vi "Plotter_Competition_Main.vi"() -> ()   [LabVIEW 2014]
doc: "Buggy_Competition Main.vi\nv4.0\nCode fior Jan 2012\n\nModified by D.Readman 1/12/2011 to 5/1/2012 \n- Replaced shift registers with FGV's.\n- Latched Switch function added.\n- Digital filtering on encoder inputs added."
uses:
  Controls/Plotter States.ctl
  <vilib>/Platform/TimedLoop/XDataNode/timing_clust.ctl
  <vilib>/Platform/TimedLoop/XDataNode/nitl_modes.ctl
  <vilib>/Platform/TimedLoop/XDataNode/wakeup.ctl
  <vilib>/FPGAPlugInAG/myRIO-1900/niLvFpga_Open_myRIO-1900.vi
  <vilib>/rvi/interface/nirviOpenFPGA/nirviOpenFPGA.xnode
  FPGA Bitfiles/Buggycompetition_FPGATarget2_AeroBuggyFPGA_9DbUQD1BP7s.lvbitx
  FPGA/FPGA.vi
  <vilib>/Platform/TimedLoop/XDataNode/XDataNode.xnode
  <vilib>/Platform/TimedLoop/XDataNode/XDNodeRunTimeDep.lvlib
panel:
  out "Array 2":i32[][](array[numeric])
  out "M2 desired":i32
  out "M1 desired":i32
  out "m2 current":i16
  out "M1 current":i16
  out "Array":dbl[][](array[numeric])
  out "Finished Late? [i-1]":bool
  in  "Sample interval":u32=100000
  in  "MWidth":i64=4
  out "Current State":T1
  out "Switch B":bool
  out "Switch A":bool
  in  "Enc. Filter":i16=2 min=0 step=1
  out "Switches Latched":cluster{"Switch A GN":bool, "Switch B BL":bool}
  in  "Terminate":bool
  out "Error Display":errorcluster
  in  "Reset Button":bool
  # "Impeccable Plotter Controller"
  # "Switches"
  # "Admin controls - Do not alter"
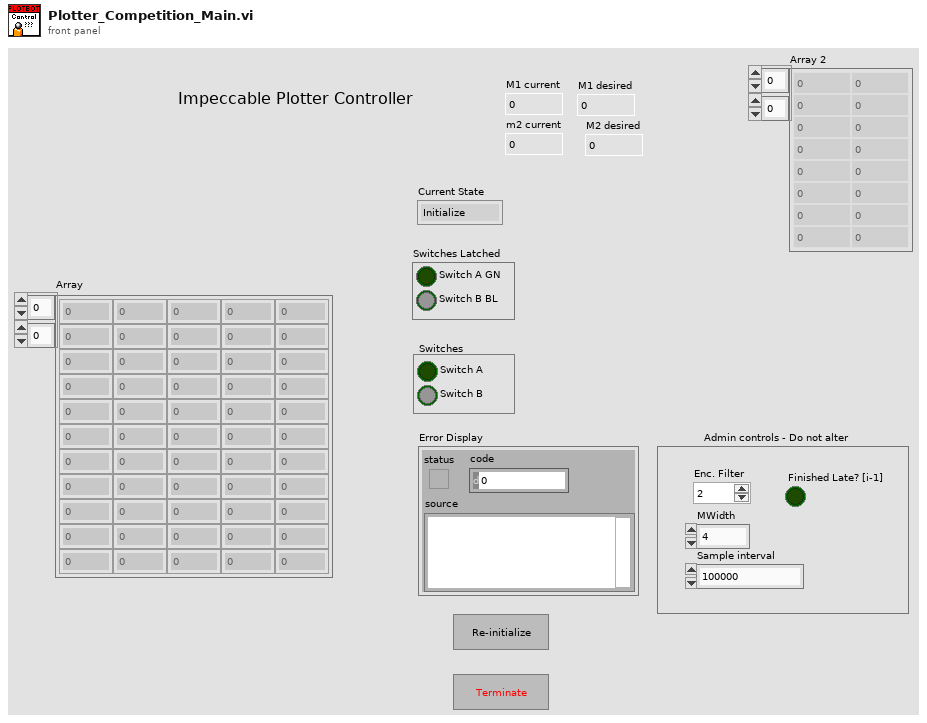
[diagram p1: front panel]
types:
  T1 = typedef "Plotter States.ctl" = enum16{"Initialize", "Run", "Stop"}
  T2 = cluster{"Data":dbl[], "Operation":enum16{"New folder/file", "Create file", "Record", "Close"}, "File name":string}
  T3 = typedef "XDNodeRunTimeDep.lvlib/timing_clust.ctl" = cluster{"Expected End [f-1]":u64, "Actual End [f-1]":u64, "Finished Late? [f-1]":bool, "Expected End [i-1]":u64, "Actual End [i-1]":u64, "Finished Late? [i-1]":bool, "Expected Start [i]":u64, "Actual Start [i]":u64, "Expected Start [f]":u64, "Actual Start [f]":u64, "Source Name":string, "Structure Name":string, "Period":i64, "Deadline":i64, "Offset":i64, "Start":i64, "Priority":i32, "Timeout":i32, "Mode":T4, "Wakeup Reason":T5, "Error":errorcluster, "Source Type":string, "Secondary Source Type":string, "Global End Time":u64, "Global Start Time":u64, "Frame Duration":u64, "Iteration Duration":u64, "Assigned CPU":i32, "I/O Scan Engine Mode":u32}
  T4 = typedef "XDNodeRunTimeDep.lvlib/nitl_modes.ctl" = enum32{"No Change", "Process missed periods, maintain original phase", "Discard missed periods, maintain original phase", "Process missed periods, ignore original phase", "Discard missed periods, ignore original phase"}
  T5 = typedef "XDNodeRunTimeDep.lvlib/wakeup.ctl" = enum32{"Normal", "Aborted", "Asynchronous wakeup", "Timing source error", "Timed loop error", "Timeout"}
  T6 = enum16{"New folder/file", "Create file", "Record", "Close"}
  T7 = cluster{"appended array":dbl[], "Operation":enum16{"New folder/file", "Create file", "Record", "Close"}, string}
  T8 = cluster{dbl[], "Operation":enum16{"New folder/file", "Create file", "Record", "Close"}, string}
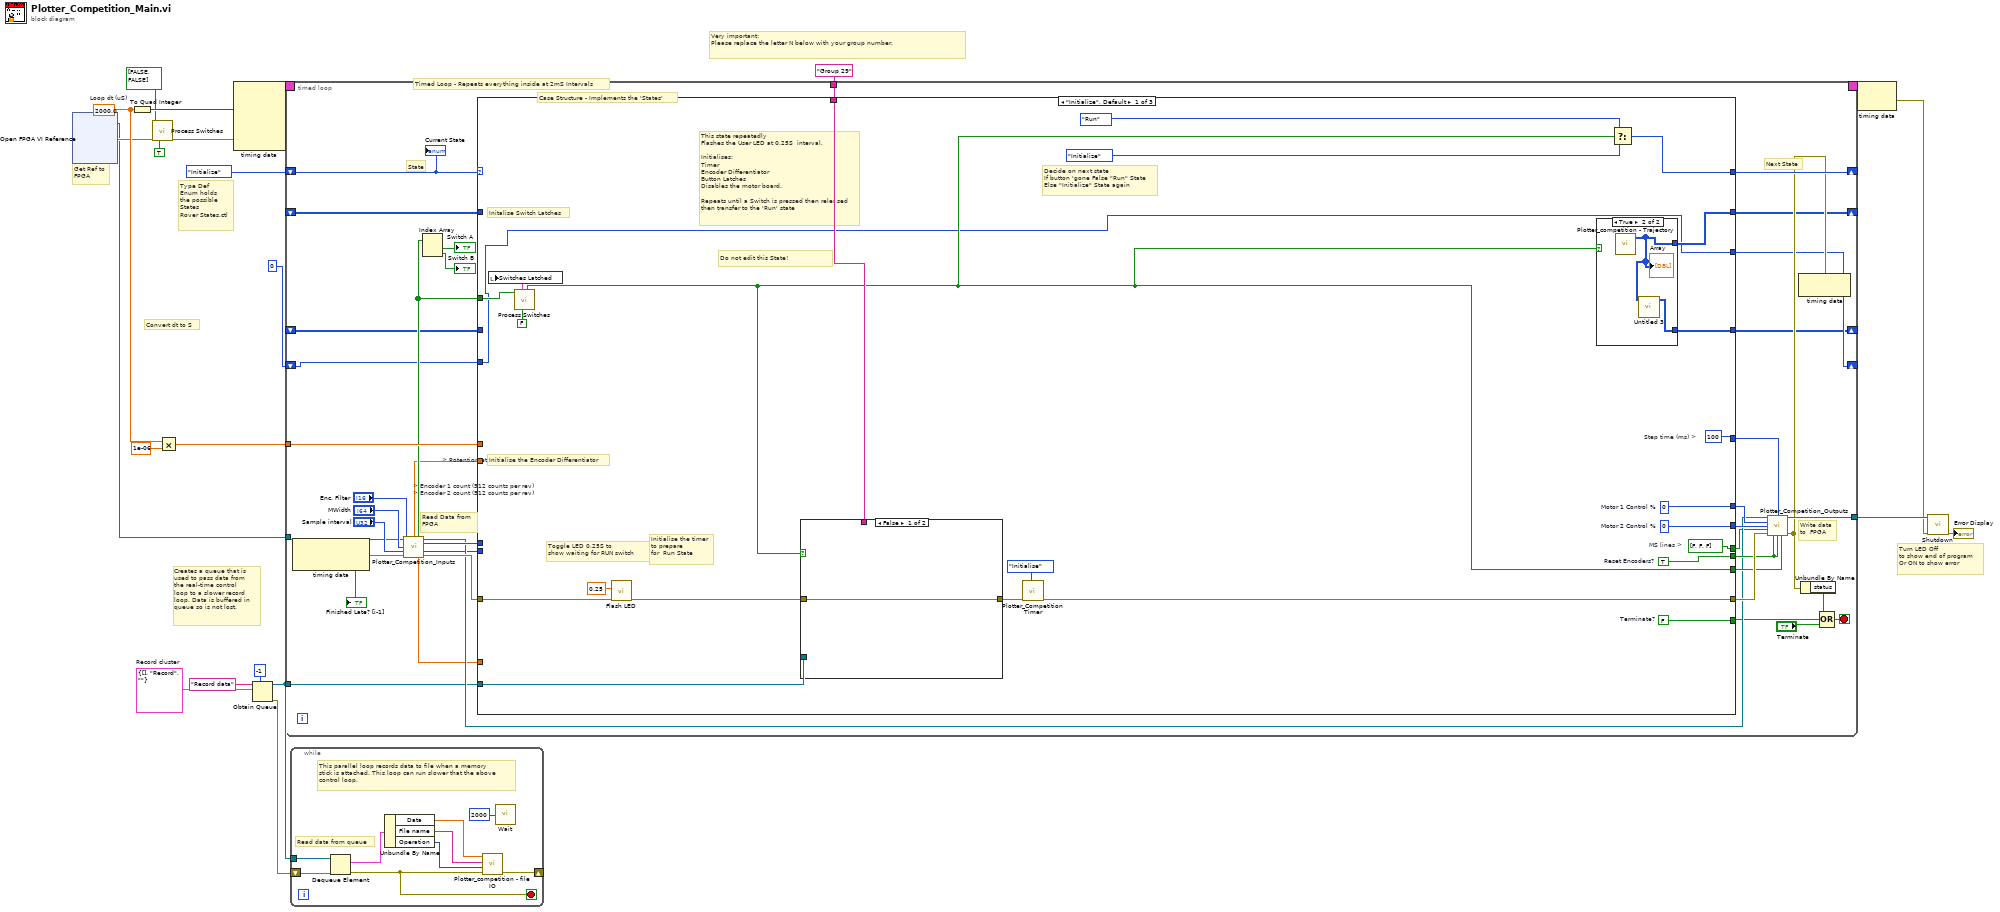
[diagram p0: block diagram]
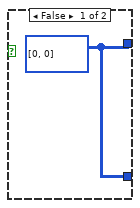
[diagram p2: hidden frame]
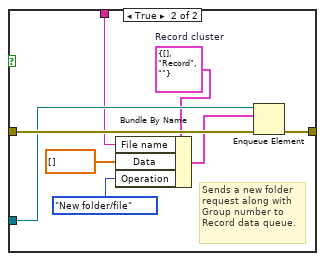
[diagram p3: hidden frame]
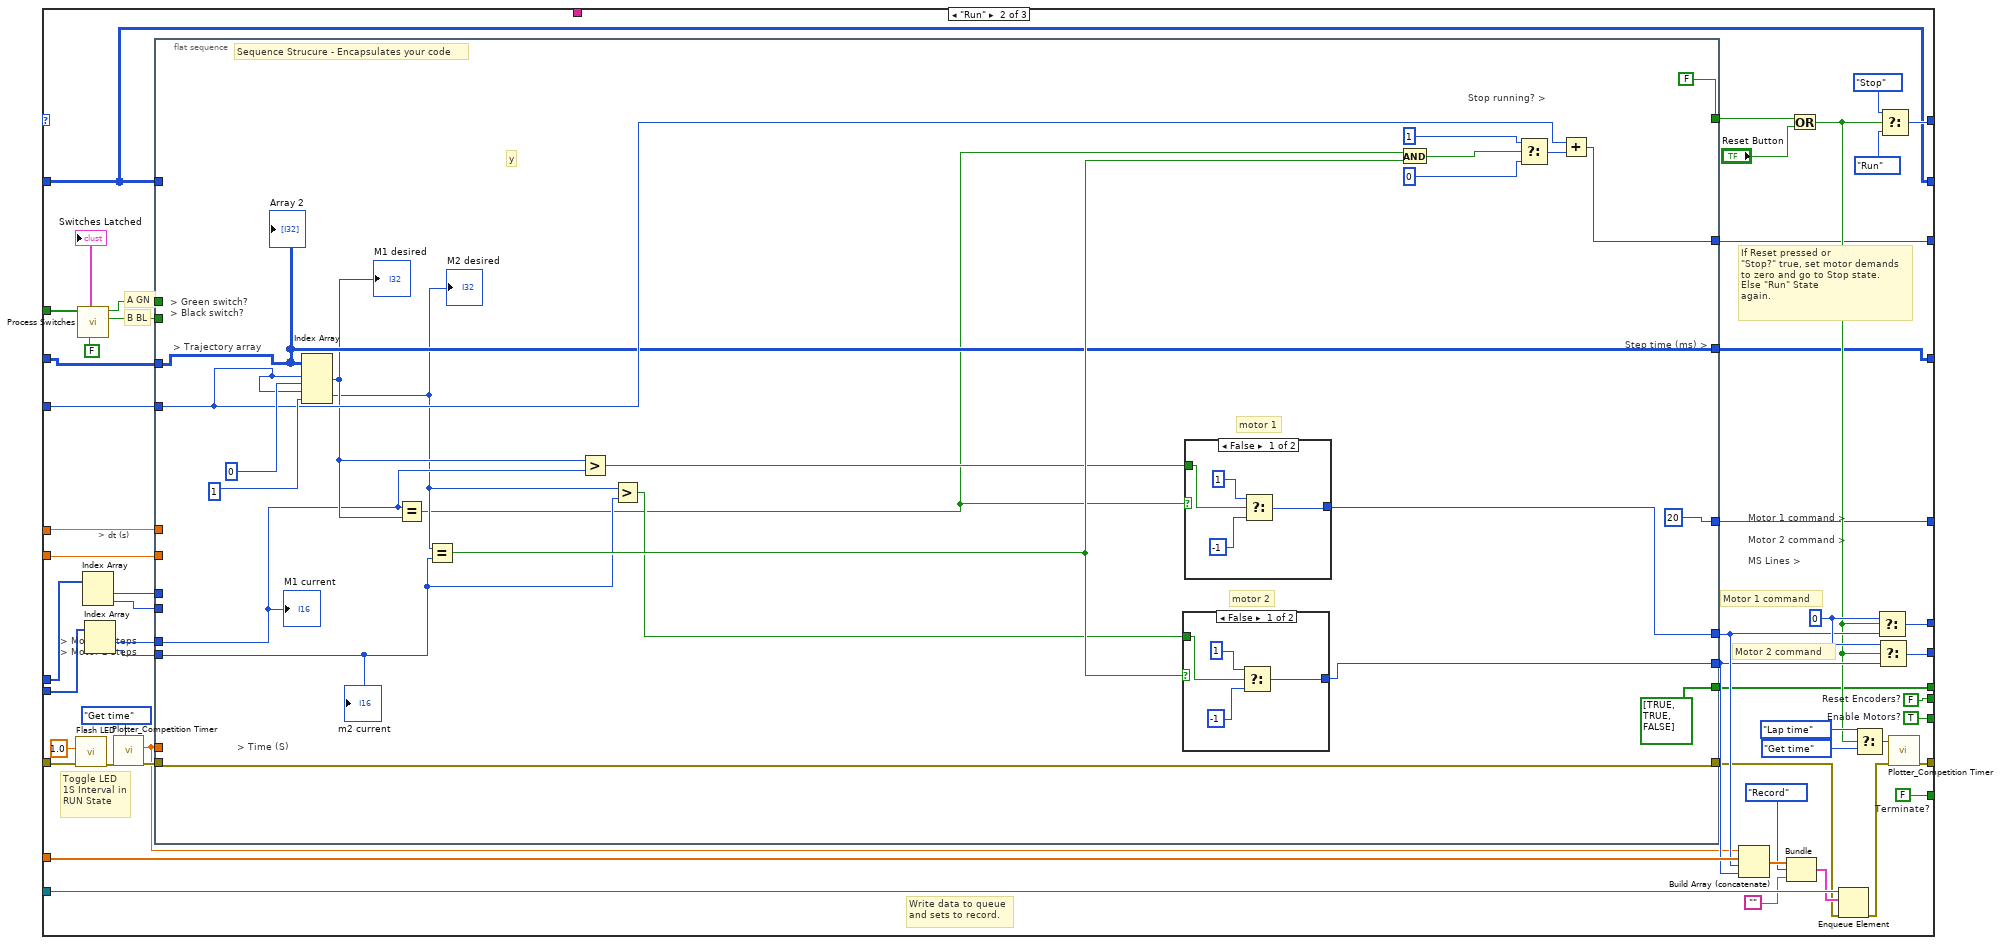
[diagram p4: hidden frame]
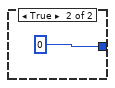
[diagram p5: hidden frame]
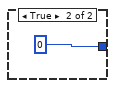
[diagram p6: hidden frame]
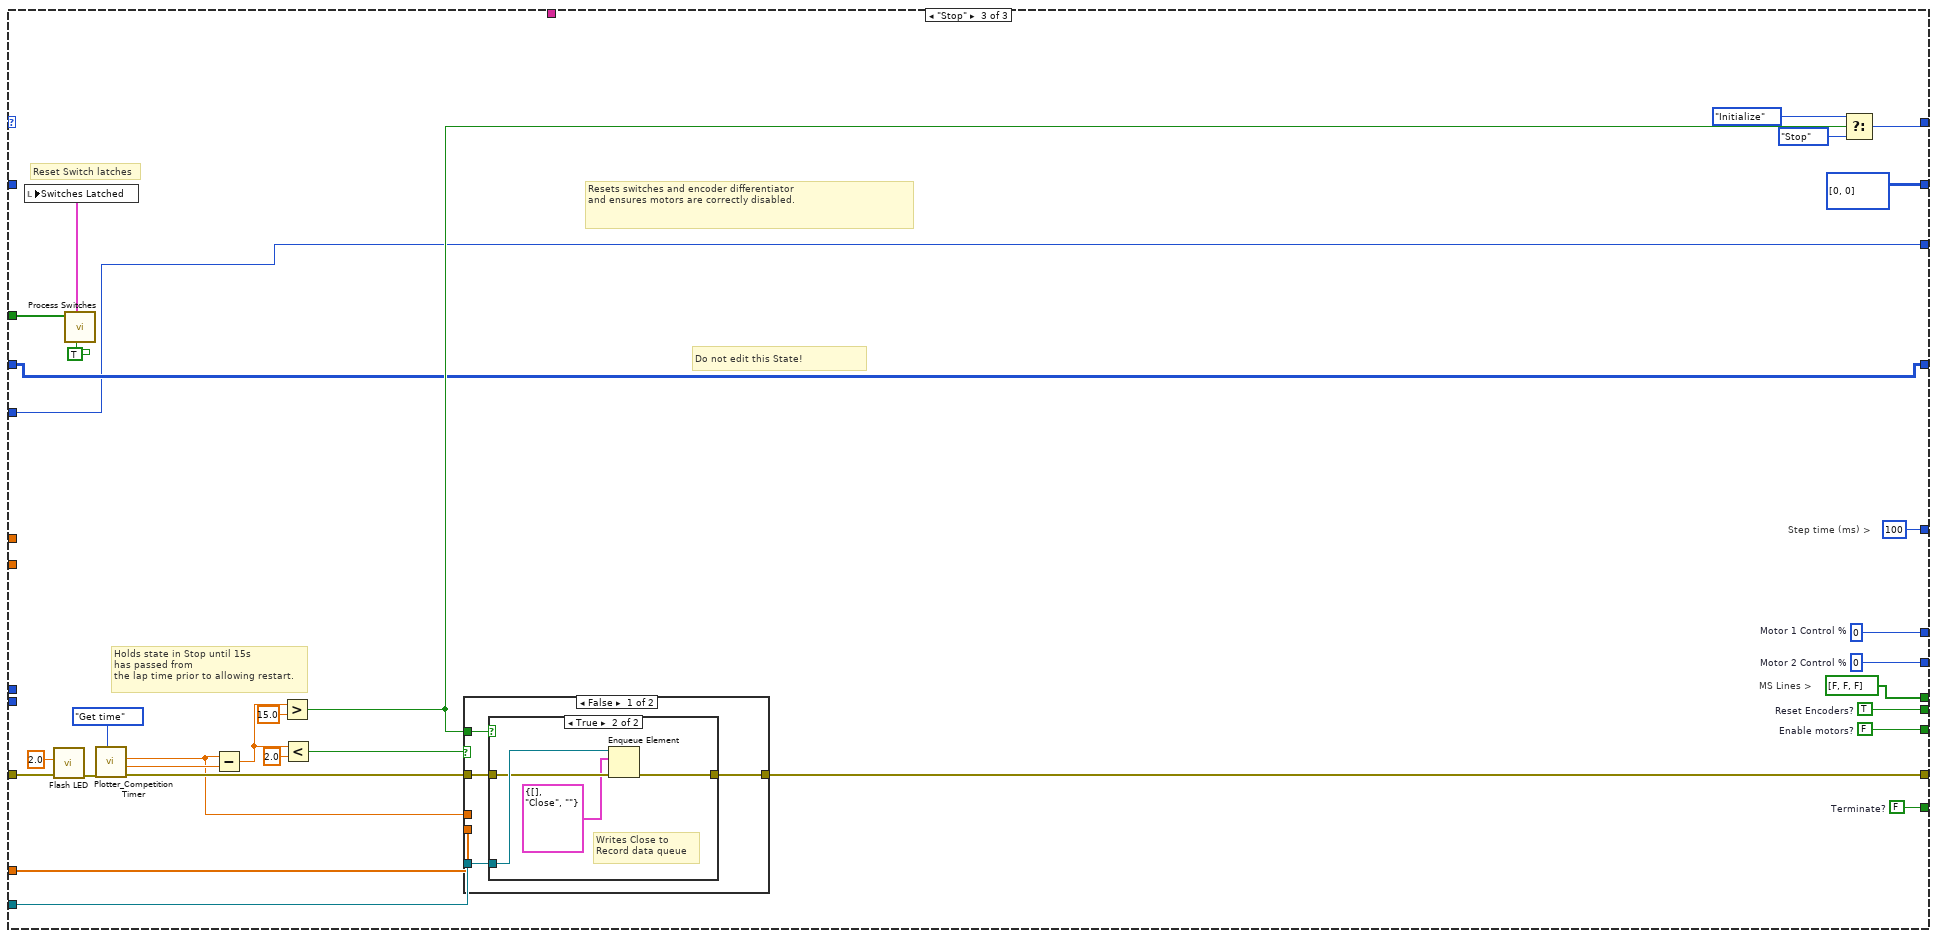
[diagram p7: hidden frame]
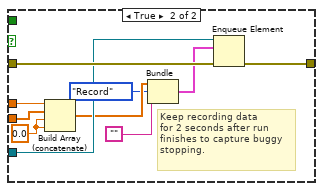
[diagram p9: hidden frame]
diagram:
  w7 = T2 {"Data"=[], "Operation"=enum."Record", "File name"=""}  # Record cluster
  w15 = 2000.0  # Loop dt (uS)
  # "Creates a queue that is\nused to pass data from\nthe real-time control \nloop to a slower record\nloop. Data is buffered in \nqueue so is not lost."
  # "Very important:\nPlease replace the letter N below with your group number."
  # "Type Def\nEnum holds\nthe possible\nStates\nRover States.ctl"
  # "Get Ref to\nFPGA"
  # "Timed Loop - Repeats everything inside at 2mS Intervals"
  # "Convert dt to S"
  # "Turn LED Off\nto show end of program\nOr ON to show error"
  n1 = xnode "Open FPGA VI Reference"() -> ("FPGA VI Reference Out"=w2:refnum<k20>, "error out"=w12:errorcluster)  [unwired: 2 in]
  n2 = To Quad Integer(1:w15) -> (0:w18:i64)
  n3 = call "Process Switches .vi"("Initialise?"=TRUE, "Error In"=w12, "Switches in"=bool[] [FALSE, FALSE]) -> ("Error Out"=w8:errorcluster)  [unwired: 4 in, 4 out]
  n4 = Multiply(x=w15, y=1e-06) -> (x*y=w13:dbl)
  n5 = node-c288(w18, w8) -> (w21:T3)  [unwired: 3 in]
  n6 = Obtain Queue(max queue size (-1, unlimited)=-1, name (unnamed)="Record data", element data type=w7) -> (queue out=w5:refnum<queue>, error out=w4:errorcluster)  [unwired: 2 in, 1 out]
  n7 = timed-loop {
    shift-right: [w60] -> _
    shift-left: Plotter_States."Initialize" ("Initial State") -> [w61]
    timing: w21 -> [_]
    timing-out: [_] -> w20
    tunnel: [w56] -> w19
    tunnel: w13 -> [w51]
    tunnel: w2 -> [w23]
    tunnel: "Group 29" -> [w39]
    tunnel: w5 -> [w33]
    shift-right: [w29] -> _
    shift-left: _ -> [w28]
    shift-right: [w27] -> _
    shift-left: 0 -> [w24]
    shift-right: [w26] -> _
    shift-left: _ -> [w25]
    stop <- w46 stop-if-true
    # "> Potentiometer bias (-1 to +1)"
    # "> Encoder 1 count (512 counts per rev)\n> Encoder 2 count (512 counts per rev)"
    # "Case Structure - Implements the 'States'"
    # "Next State"
    # "Write data\nto  FPGA"
    # "Read Data from\nFPGA"
    # "State"
    n8 = node-c288() -> (w49:errorcluster, →"Finished Late? [i-1]":bool)  [unwired: 1 in]
    n9 = call "Plotter_Competition_Inputs.vi"("FPGA VI Reference"=w23, "Filter Iterations"="Enc. Filter", "Measurement Width (Counts)"="MWidth", "Max sample interval (uS)"="Sample interval", "Error In"=w49) -> ("Bias (-1 to +1)"=w32:dbl, "Switches Green or Black"=w36:bool[], "FPGA VI Reference Out"=w50:refnum<k20>, "Encoder count"=w59:i64[], "Motor Steps"=w40:i16[], "Data array"=w35:dbl[], "Error Out"=w58:errorcluster)  [unwired: 3 in, 1 out]
    n10 = Index Array(array=w36) -> (element #1=→"Switch A":bool, element #2=→"Switch B":bool)  [unwired: 2 in]
    n11 = case shown="\"Initialize\", Default" w61 {
      tunnel: [w91 w155 w211] -> w60
      tunnel: [w90 w151 w215] -> w47
      tunnel: w59 -> [_ w112 _]
      tunnel: w58 -> [w76 w116 w196]
      tunnel: [w79 w139 w207] -> w57
      tunnel: [w71 w152 w216] -> w55
      tunnel: [w89 w153 w217] -> w54
      tunnel: [w88 w147 w218] -> w53
      tunnel: [w87 w146 w219] -> w52
      tunnel: w51 -> [_ w140 _]
      tunnel: w40 -> [_ w135 _]
      tunnel: w39 -> [w82 _ _]
      tunnel: w36 -> [w81 w138 w205]
      tunnel: w35 -> [_ w132 w201]
      tunnel: w33 -> [w78 w128 w204]
      tunnel: w32 -> [_ w111 _]
      tunnel: [bool[] [FALSE, FALSE, FALSE] ("MS lines") w110 bool[] [FALSE, FALSE, FALSE] ("MS lines")] -> w31
      tunnel: [u32 100 ("Step time") w109 u32 100 ("Step time")] -> w30
      tunnel: [w70 w108 i32[][] [[0, 0]] ("Array")] -> w29
      tunnel: w28 -> [_ w108 _]
      tunnel: [w68 w107 w189] -> w27
      tunnel: [w69 w104 w190] -> w26
      tunnel: w25 -> [_ w106 w190]
      tunnel: w24 -> [w68 w105 w189]
      frame "Initialize", Default {
        w87 = i8 0  # Motor 2 Control %
        w88 = i8 0  # Motor 1 Control %
        w89 = TRUE  # Reset Encoders?
        w90 = FALSE  # Terminate?
        # "MS lines >"
        # "Step time (ms) >"
        # "Initalise Switch Latches"
        # "Initialise the Encoder Differentiator"
        # "This state repeatedly\nFlashes the User LED at 0.25S  interval.\n\nInitialises:\nTimer\nEncoder Differentiator\nButton Latches\nDisables the motor board.\n\nRepeats until a Switch is pressed then released\nthen transfer to the 'Run' state"
        # "Initialise the timer\nto prepare\nfor  Run State"
        # "Toggle LED 0.25S to\nshow waiting for RUN switch"
        # "Do not edit this State!"
        # "Decide on next state\nIf button 'gone False \"Run\" State\nElse \"Initialize\" State again"
        n12 = call "Process Switches .vi"("Initialise?"=FALSE, "Switches in"=w81) -> ("Switch Released?"=w71:bool, "Switches Latched Cluster"=w85:cluster{"Switch A GN":bool, "Switch B BL":bool})  [unwired: 5 in, 3 out]
        n13 = local write "Switches Latched"(w85) -> ()
        n14 = call "Flash LED.vi"("Error In"=w76, "Interval (S) (1 S)"=0.25) -> ("Error Out"=w75:errorcluster)  [unwired: 8 in, 1 out]
        n15 = case shown="False" w71 {
          tunnel: w75 -> [w95 w103]
          tunnel: [w95 w102] -> w80
          tunnel: w82 -> [_ w98]
          tunnel: w78 -> [_ w101]
          frame False {
          }
          frame True {
            w99 = T2 {"Data"=[], "Operation"=enum."Record", "File name"=""}  # Record cluster
            # "Sends a new folder\nrequest along with\nGroup number to \nRecord data queue."
            n16 = Bundle By Name(cluster=w99, "File name"=w98, "Data"=dbl[] [] ("appended array"), "Operation"=T6."New folder/file") -> (w100:T2)
            n17 = Enqueue Element(queue=w101, element=w100, error in (no error)=w103) -> (error out=w102:errorcluster)  [unwired: 1 in, 2 out]
          }
        }
        n18 = call "Plotter_Competition Timer.vi"("Timer state"=enum16{"Initialise", "Get time", "Lap time"}."Initialise", "Error In"=w80) -> ("Error Out"=w79:errorcluster)  [unwired: 7 in, 2 out]
        n19 = case shown="True" w71 {
          tunnel: [w92 w94] -> w70
          tunnel: [w92 w93] -> w69
          frame False {
            w92 = i32[][] [[0, 0]] ("Array")
          }
          frame True {
            n20 = call "Plotter_competition - Trajectory.vi"() -> ("Array"=w94:i32[][])  [unwired: 11 in]
            "Array" <- w94
            n21 = call "Untitled 3.vi"("Array"=w94) -> ("Array 2"=w93:i32[][])  [unwired: 10 in]
          }
        }
        n22 = Select(t=Plotter_States."Run" ("Buggy State"), s=w71, f=Plotter_States."Initialize" ("Buggy State")) -> (s? t:f=w91:T1)
      }
      frame "Run" {
        w145 = i8 0 ("t")
        w151 = FALSE  # Terminate?
        w152 = TRUE  # Enable Motors?
        w153 = FALSE  # Reset Encoders?
        # "Motor 1 command >\n\nMotor 2 command >\n\nMS Lines >"
        # "> dt (s)"
        # "> Motor 1 steps\n> Motor 2 steps"
        # "Write data to queue\nand sets to record."
        # "If Reset pressed or\n\"Stop?\" true, set motor demands\nto zero and go to Stop state.\nElse \"Run\" State\nagain."
        # "B BL"
        # "A GN"
        # "Sequence Strucure - Encapsulates your code"
        # "Motor 2 command"
        # "Motor 1 command"
        # "Toggle LED\n1S Interval in\nRUN State"
        n23 = call "Flash LED.vi"("Error In"=w116, "Interval (S) (1 S)"=1.0) -> ("Error Out"=w115:errorcluster)  [unwired: 8 in, 1 out]
        n24 = call "Process Switches .vi"("Initialise?"=FALSE, "Switches in"=w138) -> ("Switch B Latched"=w149:bool, "Switch A Latched"=w150:bool, "Switches Latched Cluster"=→"Switches Latched":cluster{"Switch A GN":bool, "Switch B BL":bool})  [unwired: 5 in, 2 out]
        n25 = Index Array(array=w112) -> (element #1=w137:i64, element #2=w136:i64)  [unwired: 2 in]
        n26 = Index Array(array=w135) -> (element #1=w134:i16, element #2=w133:i16)  [unwired: 2 in]
        n27 = call "Plotter_Competition Timer.vi"("Timer state"=enum16{"Initialise", "Get time", "Lap time"}."Get time", "Error In"=w115) -> ("Error Out"=w154:errorcluster, "Elapsed Time Out (S)"=w129:dbl)  [unwired: 7 in, 1 out]
        n28 = flat-sequence {
          tunnel: [w169] -> w131
          tunnel: [w165] -> w130
          tunnel: w154 -> [w178]
          tunnel: [w178] -> w124
          tunnel: w129 -> [_]
          tunnel: w150 -> [_]
          tunnel: w149 -> [_]
          tunnel: w140 -> [_]
          tunnel: w137 -> [_]
          tunnel: w136 -> [_]
          tunnel: w134 -> [w161]
          tunnel: w133 -> [w159]
          tunnel: [FALSE ("Stop")] -> w113
          tunnel: w111 -> [_]
          tunnel: [bool[] [TRUE, TRUE, FALSE] ("MS lines")] -> w110
          tunnel: [u32 20 ("Step time")] -> w109
          tunnel: w108 -> [_]
          tunnel: [w170] -> w107
          tunnel: w106 -> [w163]
          tunnel: w105 -> [w166]
          tunnel: [w163] -> w104
          frame #0 {
            # "motor 2"
            # "motor 1"
            # "> Trajectory array"
            # "y"
            # "> Green switch?\n> Black switch?"
            # "Step time (ms) >"
            # "Stop running? >"
            # "> Time (S)"
            n29 = Index Array(array=w163, index (row) #1=w166, index (col) #1=0, index (row) #2=w166, index (col) #2=1) -> (element #1=w162:i32, element #2=w160:i32)
            "M1 desired" <- w162
            "M2 desired" <- w160
            n30 = Equal?(x=w161, y=w162) -> (x = y?=w156:bool)
            n31 = Equal?(x=w160, y=w159) -> (x = y?=w164:bool)
            n32 = Greater?(x=w162, y=w161) -> (0:w158:bool)
            n33 = Greater?(x=w160, y=w159) -> (0:w157:bool)
            n34 = case shown="False" w164 {
              tunnel: [w182 0] -> w165
              tunnel: w157 -> [w179 _]
              frame False {
                n35 = Select(t=1, s=w179, f=-1) -> (s? t:f=w182:i32)
              }
              frame True {
              }
            }
            n36 = case shown="False" w156 {
              tunnel: [w187 0] -> w169
              tunnel: w158 -> [w184 _]
              frame False {
                n37 = Select(t=1, s=w184, f=-1) -> (s? t:f=w187:i32)
              }
              frame True {
              }
            }
            n38 = And(x=w156, y=w164) -> (x .and. y?=w174:bool)
            n39 = Select(t=1, s=w174, f=0) -> (s? t:f=w171:i32)
            n40 = Add(x=w166, y=w171) -> (x+y=w170:i32)
            "M1 current" <- w161
            "m2 current" <- w159
            "Array 2" <- w163
          }
        }
        n41 = Build Array (concatenate)(w129, w132, w131, w130) -> (w126:dbl[])
        n42 = Bundle(w126, "Operation"=T6."Record", "") -> (w127:T8)  [unwired: 1 in]
        n43 = Or(x=w113, y="Reset Button") -> (x .or. y?=w118:bool)
        n44 = Enqueue Element(queue=w128, element=w127, error in (no error)=w124) -> (error out=w123:errorcluster)  [unwired: 1 in, 2 out]
        n45 = Select(t=enum16{"Initialise", "Get time", "Lap time"}."Lap time" ("Timer state"), s=w118, f=enum16{"Initialise", "Get time", "Lap time"}."Get time" ("Timer state")) -> (s? t:f=w120:enum16{"Initialise", "Get time", "Lap time"})
        n46 = Select(t=w145, s=w118, f=w131) -> (s? t:f=w147:i32)
        n47 = Select(t=w145, s=w118, f=w130) -> (s? t:f=w146:i32)
        n48 = Select(t=Plotter_States."Stop" ("Buggy State"), s=w118, f=Plotter_States."Run" ("Buggy State")) -> (s? t:f=w155:T1)
        n49 = call "Plotter_Competition Timer.vi"("Timer state"=w120, "Error In"=w123) -> ("Error Out"=w139:errorcluster)  [unwired: 7 in, 2 out]
      }
      frame "Stop" {
        w215 = FALSE  # Terminate?
        w216 = FALSE  # Enable motors?
        w217 = TRUE  # Reset Encoders?
        w218 = i8 0  # Motor 1 Control %
        w219 = i8 0  # Motor 2 Control %
        # "MS Lines >"
        # "Step time (ms) >"
        # "Holds state in Stop until 15s\nhas passed from\nthe lap time prior to allowing restart."
        # "Resets switches and encoder differentiator\nand ensures motors are correctly disabled."
        # "Do not edit this State!"
        # "Reset Switch latches"
        n50 = call "Flash LED.vi"("Error In"=w196, "Interval (S) (1 S)"=2.0) -> ("Error Out"=w195:errorcluster)  [unwired: 8 in, 1 out]
        n51 = call "Process Switches .vi"("Initialise?"=TRUE, "Switches in"=w205) -> ("Switches Latched Cluster"=w213:cluster{"Switch A GN":bool, "Switch B BL":bool})  [unwired: 5 in, 4 out]
        n52 = local write "Switches Latched"(w213) -> ()
        n53 = call "Plotter_Competition Timer.vi"("Timer state"=enum16{"Initialise", "Get time", "Lap time"}."Get time", "Error In"=w195) -> ("Error Out"=w208:errorcluster, "Lap time out (s)"=w199:dbl, "Elapsed Time Out (S)"=w197:dbl)  [unwired: 7 in]
        n54 = Subtract(x=w197, y=w199) -> (x-y=w198:dbl)
        n55 = Greater?(x=w198, y=15.0) -> (0:w206:bool)
        n56 = Less?(x=w198, y=2.0) -> (x < y?=w202:bool)
        n57 = case shown="False" w202 {
          tunnel: w208 -> [w223 w238]
          tunnel: [w222 w237] -> w207
          tunnel: w206 -> [w221 _]
          tunnel: w204 -> [w220 w236]
          tunnel: w201 -> [_ w230]
          tunnel: w197 -> [_ w235]
          frame False {
            n58 = case shown="True" w221 {
              tunnel: w223 -> [w224 w227]
              tunnel: [w224 w226] -> w222
              tunnel: w220 -> [_ w228]
              frame False {
              }
              frame True {
                # "Writes Close to \nRecord data queue"
                n59 = Enqueue Element(queue=w228, element=T7 {"appended array"=[], "Operation"=enum."Close", ""}, error in (no error)=w227) -> (error out=w226:errorcluster)  [unwired: 1 in, 2 out]
              }
            }
          }
          frame True {
            w229 = 0.0 ("y")
            # "Keep recording data\nfor 2 seconds after run\nfinishes to capture buggy\nstopping."
            n60 = Build Array (concatenate)(w235, w230, w229, w229) -> (w234:dbl[])
            n61 = Bundle(w234, "Operation"=T6."Record", "") -> (w231:T8)  [unwired: 1 in]
            n62 = Enqueue Element(queue=w236, element=w231, error in (no error)=w238) -> (error out=w237:errorcluster)  [unwired: 1 in, 2 out]
          }
        }
        n63 = Select(t=Plotter_States."Initialize" ("Buggy State"), s=w206, f=Plotter_States."Stop") -> (s? t:f=w211:T1)
      }
    }
    n64 = call "Plotter_Competition_Outputs.vi"("FPGA VI Reference"=w50, "Step time"=w30, "Motor 1 command"=w53, "Motor 2 command"=w52, "MS lines"=w31, "Error In"=w57, "Reset encoder 1?"=w54, "Reset encoder 2?"=w54, "Enable motors?"=w55) -> ("FPGA VI Reference out"=w56:refnum<k20>, "Error Out"=w44:errorcluster)  [unwired: 5 in]
    n65 = node-c288(w44) -> ()  [unwired: 1 out]
    n66 = Unbundle By Name(w44) -> ("status"=w48:bool)
    n67 = Compound Arithmetic op=OR(w48, w47, "Terminate") -> (w46:bool)
    "Current State" <- w61
  }
  n68 = while {
    tunnel: w5 -> [w247]
    shift-right: [w242] -> _
    shift-left: w4 -> [w246]
    stop <- w243 stop-if-true
    # "Read data from queue"
    # "This parallel loop records data to file when a memory\nstick is attached. This loop can run slower that the above\ncontrol loop."
    n69 = Dequeue Element(queue=w247, error in (no error)=w246) -> (element=w245:T2, error out=w243:errorcluster)  [unwired: 1 in, 2 out]
    n70 = Unbundle By Name(w245) -> ("Data"=w244:dbl[], "File name"=w240:string, "Operation"=w239:T6)
    n71 = call "Plotter_competition - file IO.vi"("error in"=w243, "Operation"=w239, "File name"=w240, "Data"=w244) -> ("error out"=w242:errorcluster)  [unwired: 7 in]
    n72 = call "Wait"("Count(uSec)"=u32 2000) -> ()  [unwired: 1 out]
  }
  n73 = node-c288(w20) -> (w17:errorcluster)
  n74 = call "Shutdown.vi"("Error"=w17, "FPGA VI Reference"=w19) -> ("Error Display"=→"Error Display":errorcluster)  [unwired: 8 in]
